vi "Stop.vi"(8 "error in (no error)":errorcluster, 11 "Instrument Base in":refnum<class "Instr Base.lvclass">) -> (0 "error out":errorcluster, 3 "Instrument Base out":refnum<class "Instr Base.lvclass">)   [LabVIEW 2023, in "HAL GOOP4.lvlib" / "Instr Base.lvclass"]
uses:
  Instr Base.lvclass
  Instr Base.lvclass/Instr Base.ctl
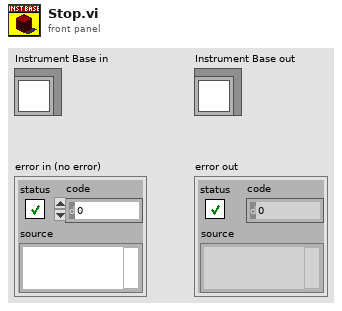
[diagram p1: front panel]
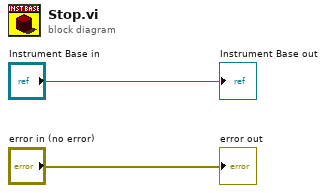
[diagram p0: block diagram]
diagram:
  "error out" <- "error in (no error)"
  "Instrument Base out" <- "Instrument Base in"
